vi "Scan Setup.vi"(8 "error in (no error)":errorcluster, 11 "Photon Counter with LCD Reader in":refnum<class "Photon Counter with LCD Reader.lvclass">) -> (0 "error out":errorcluster, 3 "Photon Counter with LCD Reader out":refnum<class "Photon Counter with LCD Reader.lvclass">)   [LabVIEW 2017, in "Photon Counter with LCD Reader.lvclass"]
doc: "(Dynamic) Send commands to configure the instrument based on the class member fields."
uses:
  Photon Counter with LCD Reader.lvclass
  Instruments/Photon Counter/SR400/Public/Typedefs.llb/Gate Mode.ctl
  Photon Counter with LCD Reader.lvclass/Photon Counter with LCD Reader.ctl
  Reader/Reader.lvclass
  Instruments/Utility Classes/Readable/Readable.lvclass
  Instruments/Photon Counter/SR400/SR400.lvlib
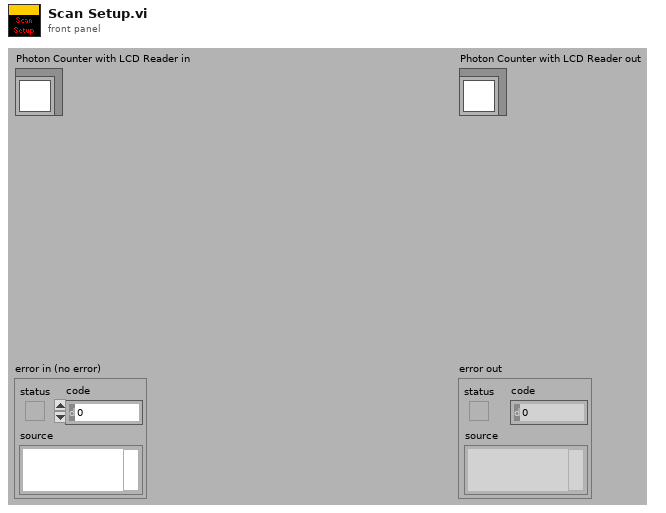
[diagram p1: front panel]
types:
  T1 = typedef "SR400.lvlib/Gate Mode.ctl" = enum16{"CW", "Fixed", "Scan"}
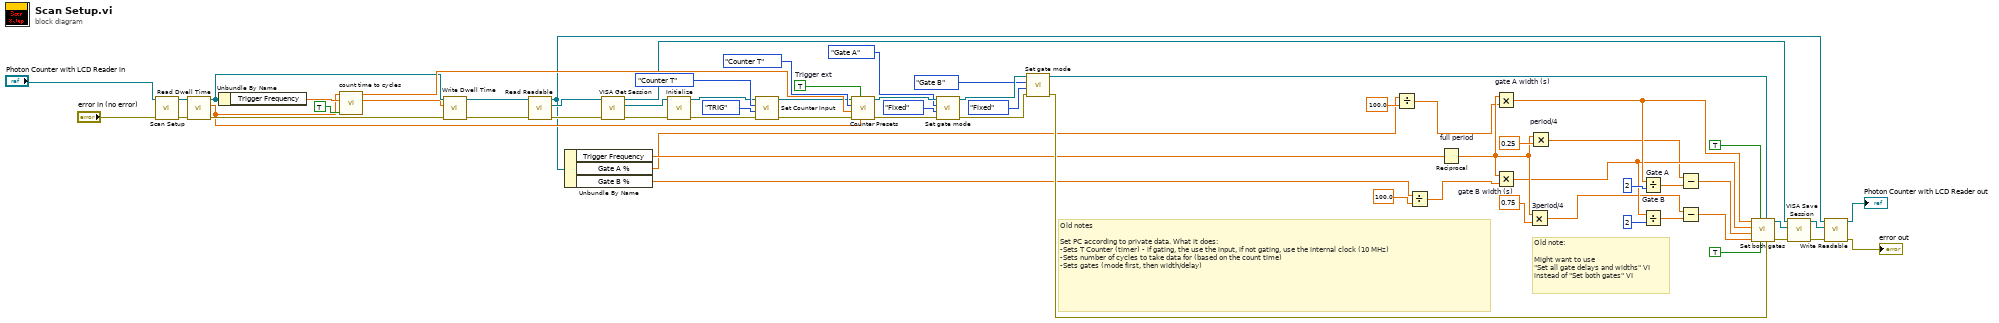
[diagram p0: block diagram]
diagram:
  w27 = TRUE  # Trigger ext
  # "Old note:\n\nMight want to use \n\"Set all gate delays and widths\" VI \ninstead of \"Set both gates\" VI"
  # "Old notes\n\nSet PC according to private data. What it does:\n-Sets T Counter (timer) - if gating, the use the input, if not gating, use the internal clock (10 MHz)\n-Sets number of cycles to take data for (based on the count time)\n-Sets gates (mode first, then width/delay)"
  n1 = call-parent "Scan Setup.vi"("error in (no error)"="error in (no error)", "Reader in"="Photon Counter with LCD Reader in") -> ("error out"=w41:errorcluster, "Reader out"=w43:refnum<class "Photon Counter with LCD Reader.lvclass">)  [unwired: 8 out]
  n2 = call-dynamic "Read Dwell Time.vi"("error in (no error)"=w41, "Reader.lvclass in"=w43) -> ("error out"=w39:errorcluster, "Dwell Time"=w30:dbl[unit], "Reader.lvclass out"=w42:refnum<class "Photon Counter with LCD Reader.lvclass">)  [unwired: 7 out]
  n3 = Unbundle By Name(w42) -> ("Trigger Frequency"=w53:dbl[unit])
  n4 = call "count time to cycles.vi"("dispmsg?"=TRUE, "Trigger Freq"=w53, "Count Time Set"=w30) -> ("Count Time Current"=w40:dbl[unit], "Number of triggers"=w52:dbl)  [unwired: 3 out]
  n5 = call-dynamic "Write Dwell Time.vi"("error in (no error)"=w39, "Dwell Time"=w40, "Reader.lvclass in"=w42) -> ("error out"=w32:errorcluster, "Reader.lvclass out"=w38:refnum<class "Photon Counter with LCD Reader.lvclass">)  [unwired: 7 out]
  n6 = call-dynamic "Read Readable.vi"("error in (no error)"=w32, "Reader.lvclass in"=w38) -> ("error out"=w33:errorcluster, "Readable.lvclass"=w31:refnum<class "Readable.lvclass">, "Reader.lvclass out"=w23:refnum<class "Photon Counter with LCD Reader.lvclass">)  [unwired: 7 out]
  n7 = Unbundle By Name(w23) -> ("Trigger Frequency"=w22:dbl[unit], "Gate A %"=w7:dbl, "Gate B %"=w4:dbl)
  n8 = call-dynamic "VISA Get Session.vi"("error in (no error)"=w33, "Instrument.lvclass in"=w31) -> ("error out"=w34:errorcluster, "VISA Resource Name"=w37:refnum<visa-resource-name>, "Instrument.lvclass out"=w46:refnum<class "Readable.lvclass">)  [unwired: 7 out]
  n9 = call "Initialize.vi"("errorIN"=w34, "VISA resource name"=w37) -> ("errorOUT"=w35:errorcluster, "VISA resource name out"=w36:refnum<visa-resource-name>)  [unwired: 8 out]
  n10 = call "Set Counter Input.vi"("error in (no error)"=w35, "Input (def: 10 MHz)"=enum16{"10 MHz", "INPUT 1", "INPUT 2", "TRIG"}."TRIG", "Counter (def: A)"=enum16{"Counter A", "Counter B", "Counter T"}."Counter T" ("i (0) 2"), "VISA resource name"=w36) -> ("error out"=w48:errorcluster, "VISA resource name out"=w47:refnum<visa-resource-name>)  [unwired: 6 out]
  n11 = call "Counter Presets.vi"("T_set"=w30, "Trigger external?"=w27, "error in (no error)"=w48, "Number of triggers"=w52, "Counter (Def: T)"=enum16{"Invalid", "Counter B", "Counter T"}."Counter T" ("i (0) 2"), "VISA resource name"=w47) -> ("error out"=w56:errorcluster, "VISA resource name out"=w59:refnum<visa-resource-name>)  [unwired: 4 out]
  n12 = call "Set gate mode.vi"("error in (no error)"=w56, "Mode (def: CW)"=Gate_Mode."Fixed", "Gate (def: A)"=enum16{"Gate A", "Gate B"}."Gate A", "VISA resource name"=w59) -> ("error out"=w57:errorcluster, "VISA resource name out"=w58:refnum<visa-resource-name>)  [unwired: 6 out]
  n13 = call "Set gate mode.vi"("error in (no error)"=w57, "Mode (def: CW)"=Gate_Mode."Fixed", "Gate (def: A)"=enum16{"Gate A", "Gate B"}."Gate B", "VISA resource name"=w58) -> ("error out"=w61:errorcluster, "VISA resource name out"=w60:refnum<visa-resource-name>)  [unwired: 6 out]
  n14 = Divide(x=w7, y=100.0) -> (x/y=w6:dbl)
  n15 = Divide(x=w4, y=100.0) -> (x/y=w3:dbl)
  n16 = Reciprocal "full period"(x=w22) -> (1/x=w19:dbl[unit])
  n17 = Multiply "gate A width (s)"(x=w19, y=w6) -> (x*y=w15:dbl[unit])
  n18 = Multiply "gate B width (s)"(x=w19, y=w3) -> (x*y=w14:dbl[unit])
  n19 = Multiply "3period/4"(x=w19, y=0.75) -> (x*y=w11:dbl[unit])
  n20 = Multiply "period/4"(x=w19, y=0.25) -> (x*y=w12:dbl[unit])
  n21 = Divide "Gate A"(x=w15, y=2) -> (x/y=w16:dbl[unit])
  n22 = Divide "Gate B"(x=w14, y=2) -> (x/y=w13:dbl[unit])
  n23 = Subtract(x=w12, y=w16) -> (x-y=w10:dbl[unit])
  n24 = Subtract(x=w11, y=w13) -> (x-y=w9:dbl[unit])
  n25 = call "Set both gates.vi"("Error In"=w61, "VISA resource name"=w60, "Set Delay?"=TRUE, "Set Width?"=TRUE, "gatedelayoffsetB"=w9, "gatedelayoffsetA"=w10, "Gate B Width"=w14, "Gate A Width"=w15) -> ("Error Out"=w62:errorcluster, "VISA resource name out"=w65:refnum<visa-resource-name>)  [unwired: 2 out]
  n26 = call-dynamic "VISA Save Session.vi"("error in (no error)"=w62, "VISA Resource Name"=w65, "Instrument.lvclass in"=w46) -> ("error out"=w44:errorcluster, "Instrument.lvclass out"=w45:refnum<class "Readable.lvclass">)  [unwired: 7 out]
  n27 = call-dynamic "Write Readable.vi"("error in (no error)"=w44, "Readable.lvclass"=w45, "Reader.lvclass in"=w23) -> ("error out"=→"error out":errorcluster, "Reader.lvclass out"=→"Photon Counter with LCD Reader out":refnum<class "Photon Counter with LCD Reader.lvclass">)  [unwired: 7 out]
